vi "Change Status.vi"(8 "error in (no error)":errorcluster, 11 "Time Protocol in":refnum<class "Time Protocol.lvclass">) -> (0 "error out":errorcluster, 3 "Time Protocol out":refnum<class "Time Protocol.lvclass">)   [LabVIEW 2013, in "Time Protocol Actor.lvlib" / "Time Protocol.lvclass"]
uses:
  Time Protocol.lvclass
  Time Protocol.lvclass/Time Protocol.ctl
  Read History.vi
  Read Code.vi
  Read Path.vi
  Read Open.vi
  Read State.vi
  <vilib>/Utility/file.llb/Read From Spreadsheet File (string).vi
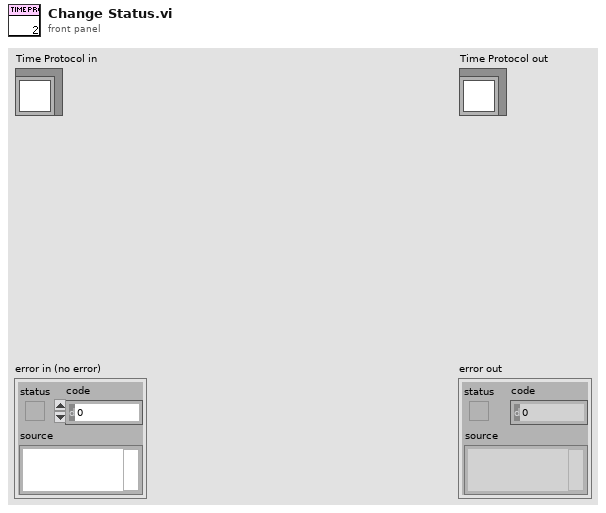
[diagram p1: front panel]
types:
  T1 = enum8{"Enabled", "Disabled", "Disabled and Grayed Out"}
  T2 = enum32{"Pause Button", "Play Button", "Media Stop Button"}
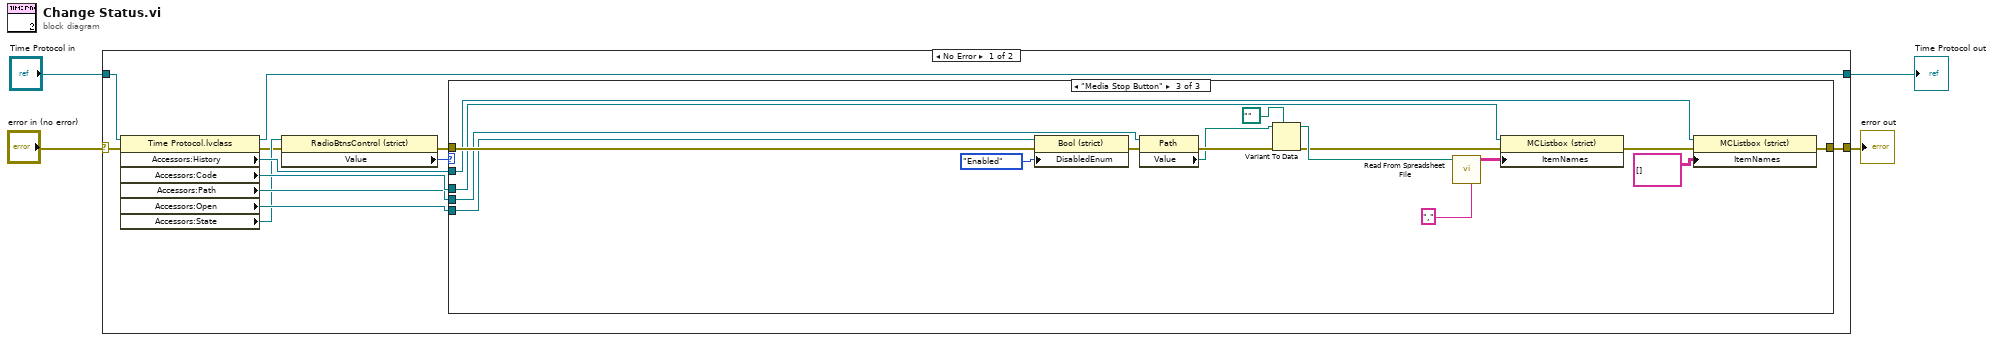
[diagram p0: block diagram]
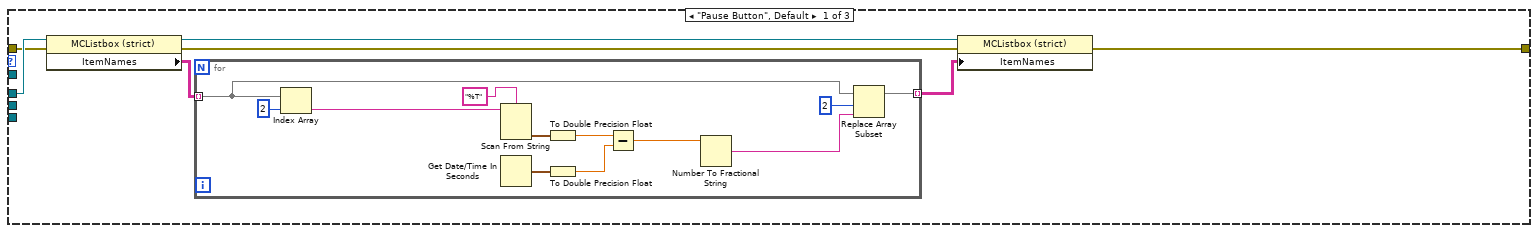
[diagram p2: hidden frame]
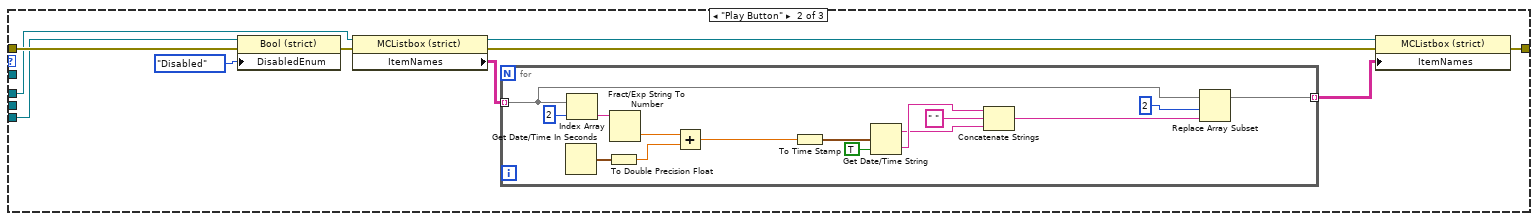
[diagram p3: hidden frame]
diagram:
  n1 = case shown="No Error" "error in (no error)" {
    selector: "error in (no error)" -> [w6 w79]
    tunnel: [w5 w79] -> w3
    tunnel: [w13 w78] -> w1
    tunnel: "Time Protocol in" -> [w14 w78]
    frame No Error {
      n2 = property class="Time Protocol.lvclass"(reference=w14, error in=w6) -> (reference out=w13:refnum<class "Time Protocol.lvclass">, error out=w7:errorcluster, "Accessors:History"=w12:refnum<vi>, "Accessors:Code"=w11:refnum<vi>, "Accessors:Path"=w10:refnum<vi>, "Accessors:Open"=w9:refnum<vi>, "Accessors:State"=w8:refnum<vi>)
      n3 = property class="RadioBtnsControl (strict)"(reference=w8, error in=w7) -> (error out=w16:errorcluster, "Value"=w15:T2)  [unwired: 1 out]
      n4 = case shown="\"Media Stop Button\"" w15 {
        tunnel: [w17 w38 w63] -> w5
        tunnel: w16 -> [w18 w45 w77]
        tunnel: w9 -> [_ w36 w61]
        tunnel: w11 -> [w19 w41 w76]
        tunnel: w10 -> [_ _ w75]
        tunnel: w12 -> [_ _ w65]
        frame "Pause Button", Default {
          n5 = property class="MCListbox (strict)"(reference=w19, error in=w18) -> (reference out=w22:refnum<vi>, error out=w23:errorcluster, "ItemNames"=w21:string[][])
          n6 = for {
            tunnel: w21 -> [w34] mode=indexing
            tunnel: [w32] -> w20 mode=indexing
            n7 = Index Array(array=w34, index=2) -> (element=w28:string)
            n8 = Scan From String(format string="%T", input string=w28) -> (output 1=w30:timestamp)  [unwired: 3 in, 3 out]
            n9 = Get Date/Time In Seconds() -> (seconds since 1Jan1904=w29:timestamp)
            n10 = To Double Precision Float(number=w30) -> (double precision float=w27:dbl)
            n11 = To Double Precision Float(number=w29) -> (double precision float=w26:dbl)
            n12 = Subtract(x=w27, y=w26) -> (x-y=w25:dbl)
            n13 = Number To Fractional String(number=w25) -> (F-format string=w24:string)  [unwired: 3 in]
            n14 = Replace Array Subset(array=w34, new element=w24, index=2) -> (w32:string[])
          }
          n15 = property class="MCListbox (strict)"(reference=w22, error in=w23, "ItemNames"=w20) -> (error out=w17:errorcluster)  [unwired: 1 out]
        }
        frame "Play Button" {
          n16 = property class="Bool (strict)"(reference=w36, error in=w45, "DisabledEnum"=T1."Disabled" ("Disabled")) -> (error out=w42:errorcluster)  [unwired: 1 out]
          n17 = property class="MCListbox (strict)"(reference=w41, error in=w42) -> (reference out=w43:refnum<vi>, error out=w44:errorcluster, "ItemNames"=w40:string[][])
          n18 = for {
            tunnel: w40 -> [w55] mode=indexing
            tunnel: [w52] -> w39 mode=indexing
            n19 = Get Date/Time In Seconds() -> (seconds since 1Jan1904=w59:timestamp)
            n20 = Index Array(array=w55, index=2) -> (element=w58:string)
            n21 = To Double Precision Float(number=w59) -> (double precision float=w56:dbl)
            n22 = Fract/Exp String To Number(string=w58) -> (number=w57:dbl)  [unwired: 3 in, 1 out]
            n23 = Add(x=w57, y=w56) -> (x+y=w53:dbl)
            n24 = To Time Stamp(1:w53) -> (0:w48:timestamp)
            n25 = Get Date/Time String(seconds (now)=w48, want seconds? (F)=TRUE) -> (date string=w50:string, time string=w51:string)  [unwired: 1 in]
            n26 = Concatenate Strings(w51, " " ("string"), w50) -> (w47:string)
            n27 = Replace Array Subset(array=w55, new element=w47, index=2) -> (w52:string[])
          }
          n28 = property class="MCListbox (strict)"(reference=w43, error in=w44, "ItemNames"=w39) -> (error out=w38:errorcluster)  [unwired: 1 out]
        }
        frame "Media Stop Button" {
          n29 = property class="Bool (strict)"(reference=w61, error in=w77, "DisabledEnum"=T1."Enabled" ("Disabled")) -> (error out=w74:errorcluster)  [unwired: 1 out]
          n30 = property class="Path"(reference=w75, error in=w74) -> (error out=w72:errorcluster, "Value"=w70:path)  [unwired: 1 out]
          n31 = Variant To Data(error in=w72, type=path "", Variant=w70) -> (data=w69:path, error out=w68:errorcluster)
          n32 = call-poly <vilib>:"Read From Spreadsheet File.vi"("delimiter (\\t)"="," ("delimiter (\\t)"), "file path (dialog if empty)"=w69) -> ("all rows"=w67:string[][])  [unwired: 5 in, 4 out]
          n33 = property class="MCListbox (strict)"(reference=w76, error in=w68, "ItemNames"=w67) -> (error out=w64:errorcluster)  [unwired: 1 out]
          n34 = property class="MCListbox (strict)"(reference=w65, error in=w64, "ItemNames"=string[][] [] ("Item Names")) -> (error out=w63:errorcluster)  [unwired: 1 out]
        }
      }
    }
    frame Error {
    }
  }
  "error out" <- w3
  "Time Protocol out" <- w1
